vi "Table-Clear column header.vi"(8 "error in (no error)":errorcluster, 11 "Table in":refnum<vi>) -> (0 "error out":errorcluster, 3 "Table out":refnum<vi>)   [LabVIEW 2017]
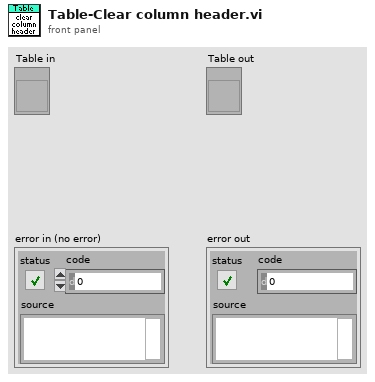
[diagram p1: front panel]
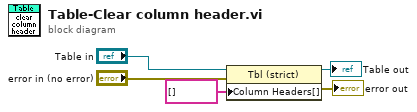
[diagram p0: block diagram]
diagram:
  n1 = property on="Property Node" class="Tbl (strict)"(reference="Table in", error in="error in (no error)", "Column Headers[]"=string[] [] ("Column Header Strings[]")) -> (reference out=→"Table out":refnum<vi>, error out=→"error out":errorcluster)
